vi "Cleanup Temp Sysdef Files.vi"(6 "bypass cleanup":bool, 8 "error in":errorcluster, 11 "Relative path":path=path "") -> (0 "error out":errorcluster)   [LabVIEW 2017, in "Routing and Faulting System Tests.lvclass"]
uses:
  Routing and Faulting System Tests.lvclass
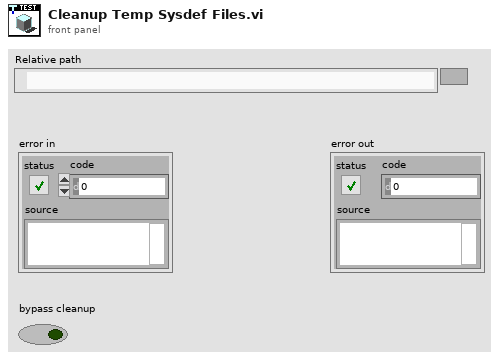
[diagram p1: front panel]
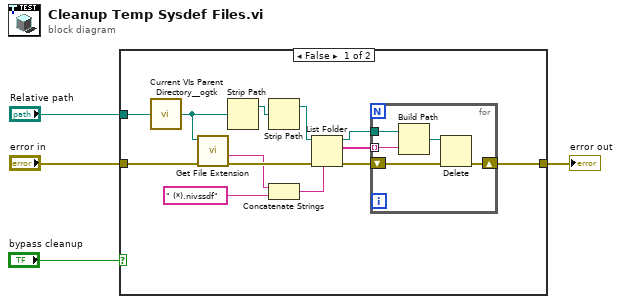
[diagram p0: block diagram]
diagram:
  n1 = case shown="False" "bypass cleanup" {
    tunnel: "Relative path" -> [w17 _]
    tunnel: "error in" -> [w12 w23]
    tunnel: [w7 w23] -> w2
    frame False {
      n2 = call <userlib>:"Current VIs Parent Directory__ogtk.vi"("Relative path (.)"=w17) -> ("Parent Directory (+ Relative)"=w5:path)  [unwired: 4 in]
      n3 = call <vilib>:"Get File Extension.vi"("error in (no error)"=w12, "file"=w5) -> ("error out"=w11:errorcluster, "filename without extension"=w10:string)  [unwired: 5 in, 3 out]
      n4 = Strip Path(path=w5) -> (stripped path=w6:path)  [unwired: 1 out]
      n5 = Strip Path(path=w6) -> (stripped path=w13:path)  [unwired: 1 out]
      n6 = Concatenate Strings(w10, " (*).nivssdf" ("pattern")) -> (w8:string)
      n7 = List Folder(path=w13, pattern=w8, error in=w11) -> (path out=w16:path, filenames=w15:string[], error out=w14:errorcluster)  [unwired: 1 in, 1 out]
      n8 = for {
        tunnel: w16 -> [w22]
        tunnel: w15 -> [w21] mode=indexing
        shift-right: [w18] -> w7
        shift-left: w14 -> [w19]
        n9 = Build Path(base path=w22, name or relative path=w21) -> (appended path=w20:path)
        n10 = Delete(path (use dialog)=w20, error in=w19) -> (error out=w18:errorcluster)  [unwired: 3 in, 2 out]
      }
    }
    frame True {
    }
  }
  "error out" <- w2
